vi "AB_820_850_Change_Path_from_Label.vi"(8 "error in (no error)":errorcluster, 9 "new label":string, 10 "old label":string, 11 "Path in":path) -> (0 "error out":errorcluster, 3 "Path out":path, 5 "changed?":bool)   [LabVIEW 2020]
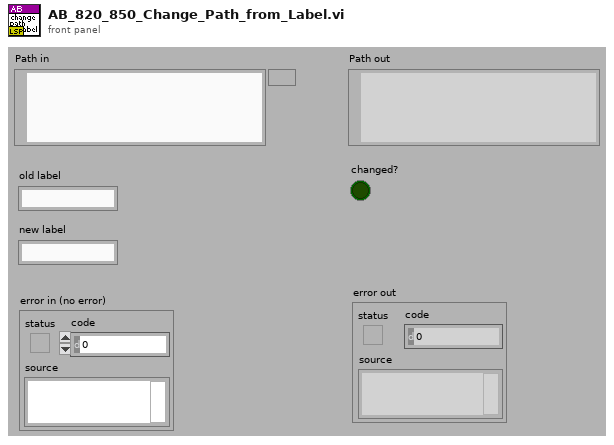
[diagram p1: front panel]
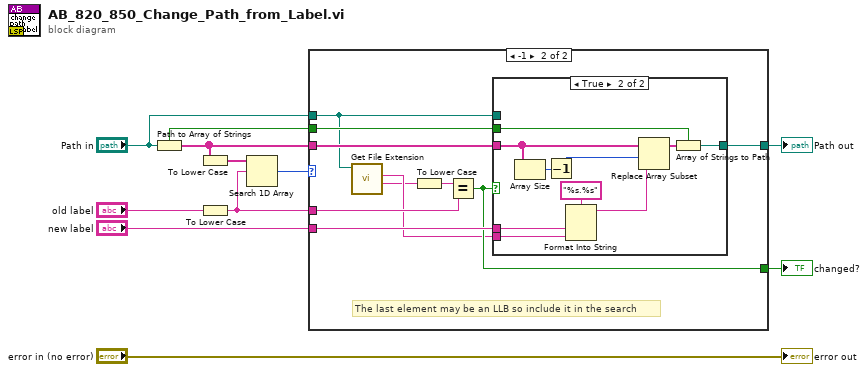
[diagram p0: block diagram]
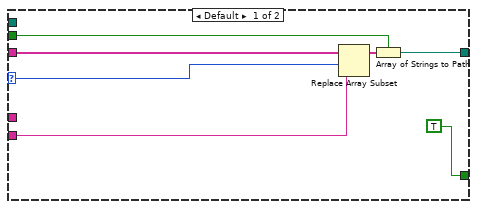
[diagram p2: hidden frame]
diagram:
  n1 = Path to Array of Strings(0:"Path in") -> (1:w11:bool, 2:w6:string[])
  n2 = To Lower Case(string=w6) -> (all lower case string=w5:string[])
  n3 = To Lower Case(string="old label") -> (all lower case string=w2:string)
  n4 = Search 1D Array(1D array=w5, element=w2) -> (index of element=w3:i32)  [unwired: 1 in]
  n5 = case shown="-1" w3 {
    selector: w3 -> [w14 _]
    tunnel: w11 -> [w17 w25]
    tunnel: "new label" -> [w13 w24]
    tunnel: w6 -> [w16 w23]
    tunnel: [w15 w26] -> w9
    tunnel: "Path in" -> [_ w21]
    tunnel: w2 -> [_ w27]
    tunnel: [TRUE w22] -> w1
    frame Default {
      n6 = Replace Array Subset(array=w16, new element=w13, index=w14) -> (w18:string[])
      n7 = Array of Strings to Path(0:w18, 1:w17) -> (2:w15:path)
    }
    frame -1 {
      # "The last element may be an LLB so include it in the search"
      n8 = call <vilib>:"Get File Extension.vi"("file"=w21) -> ("filename without extension"=w19:string, "lowercase file extension"=w20:string)  [unwired: 6 in, 3 out]
      n9 = To Lower Case(string=w19) -> (all lower case string=w28:string)
      n10 = Equal?(x=w28, y=w27) -> (x = y?=w22:bool)
      n11 = case shown="True" w22 {
        tunnel: [w29 w38] -> w26
        tunnel: w25 -> [_ w37]
        tunnel: w20 -> [_ w30]
        tunnel: w24 -> [_ w32]
        tunnel: w23 -> [_ w36]
        tunnel: w21 -> [w29 _]
        frame False {
        }
        frame True {
          n12 = Array Size(array=w36) -> (size(s)=w35:i32)
          n13 = Decrement(x=w35) -> (x-1=w34:i32)
          n14 = Format Into String(format string="%s.%s", w32, w30) -> (resulting string=w31:string)  [unwired: 2 in, 1 out]
          n15 = Replace Array Subset(array=w36, new element=w31, index=w34) -> (w39:string[])
          n16 = Array of Strings to Path(0:w39, 1:w37) -> (2:w38:path)
        }
      }
    }
  }
  "Path out" <- w9
  "changed?" <- w1
  "error out" <- "error in (no error)"
